vi "氨氮通讯.vi"() -> ()   [LabVIEW 2016, in "斯坦道氨氮.lvlib"]
uses:
  <vilib>/Plasmionique/MB Master/MB_Master_TCP/MB_Master_TCP.lvclass
  C:/Program Files (x86)/National Instruments/LabVIEW 2016/vi.lib/Plasmionique/MB Master/MB_Master/MB_Master.lvclass
  <vilib>/NI/Modbus Library/API/Wrapper/Create TCP Slave.vi
  <vilib>/Utility/config.llb/Write Key (String).vi
  <vilib>/Plasmionique/MB Master/MB_Master/MB_Master.lvclass
  <vilib>/NI/Modbus Library/API/slave/Modbus Slave.lvclass
  <vilib>/Utility/config.llb/NI_LVConfig.lvlib
  <vilib>/Plasmionique/MB Master/MB Master.lvlib
  <vilib>/NI/Modbus Library/API/Wrapper/API Main.lvlib
panel:
  out "测量数据区":T1 {"单位" items=["ug/L", "mg/L", "ppm", "mg/m3", "cm", "ppb", "ug/m3", "%", "nmol/mol", "umol/mol", "MPN/L", "MPN/100ml", "ng/m3", "NTU", "无量纲", "ms/cm", "us/cm", "℃", "mV", "万个/L"]}
  out "状态告警区":u16[](array[numeric])
  out "测量数据区":u16[](array[numeric])
  out "序列号":string
  out "状态告警区":T2
  out "status":bool
  out "关键参数区":T3
  in  "读关键参数区":bool
  in  "读状态告警区":bool
  in  "读测量数据区":bool
  in  "站号":u16(ring) items=["总磷"=1, "氨氮"=3]
  in  "停止":bool
  in  "启动":bool
  in  "控制命令":u16(ring) items=["启动测量"=1, "标样核查"=2, "零点核查"=3, "跨度核查"=4, "空白测试"=5, "平行样测试"=6, "加标回收"=7, "空白校准"=8, "标样校准"=9, "初始化（清洗）"=10, "停止测试"=11, "仪器重启"=12, "校时"=13, "模式设置"=14, "测量间隔设置"=15]
  in  "控制命令参数":u16[](array[numeric]) format="%04xH"
  in  "VISA Resource":refnum<visa-resource-name>
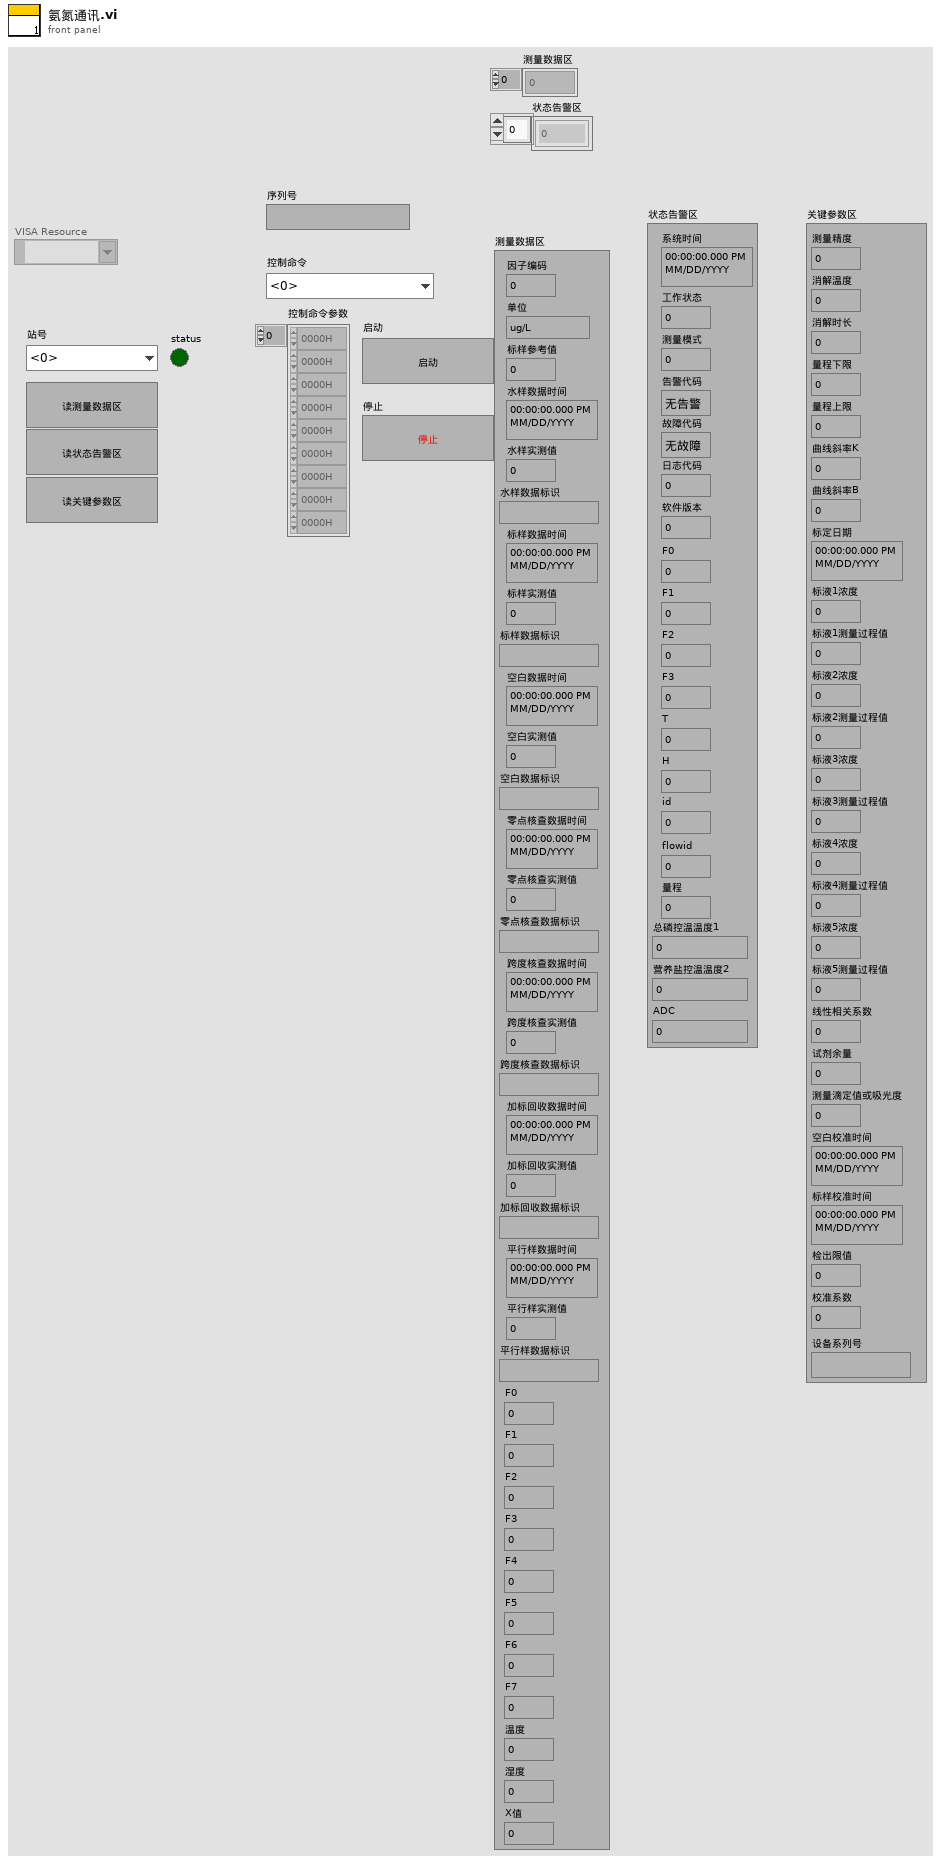
[diagram p1: front panel]
types:
  T1 = cluster{"因子编码":u32, "单位":u16, "标样参考值":sgl, "水样数据时间":timestamp, "水样实测值":sgl, "水样数据标识":string, "标样数据时间":timestamp, "标样实测值":sgl, "标样数据标识":string, "空白数据时间":timestamp, "空白实测值":sgl, "空白数据标识":string, "零点核查数据时间":timestamp, "零点核查实测值":sgl, "零点核查数据标识":string, "跨度核查数据时间":timestamp, "跨度核查实测值":sgl, "跨度核查数据标识":string, "加标回收数据时间":timestamp, "加标回收实测值":sgl, "加标回收数据标识":string, "平行样数据时间":timestamp, "平行样实测值":sgl, "平行样数据标识":string, "F0":sgl, "F1":sgl, "F2":sgl, "F3":sgl, "F4":sgl, "F5":sgl, "F6":sgl, "F7":sgl, "温度":sgl, "湿度":sgl, "X值":sgl}
  T2 = cluster{"系统时间":timestamp, "工作状态":u16, "测量模式":u16, "告警代码":enum16{"无告警", "缺试剂告警", "缺水样告警", "缺蒸馏水告警", "缺标液告警", "仪表漏液告警", "标定异常告警", "超量程告警", "加热异常", "低试剂预警", "超上限告警", "超下限告警", "仪表内部其他异常", "滴定异常告警", "电极异常告警", "量程切换告警", "参数设置告警", "PH电极电位异常", "电导率电极异常", "浊度光度异常", "溶解氧电极异常", "溶解氧光强异常", "温度异常告警", "PH异常告警", "溶解氧异常告警", "电导率异常告警", "浊度异常告警", "叶绿素异常告警", "藻密度异常告警", "蓝绿藻异常告警", "ORP异常告警", "氨氮异常告警", "清洁刷异常告警", "SD卡异常告警", "蓝牙异常告警", "Wifi异常告警", "流程异常告警"}, "故障代码":enum16{"无故障", "电机故障", "温度故障", "通讯故障", "滴定故障"}, "日志代码":u16, "软件版本":u16, "F0":sgl, "F1":sgl, "F2":sgl, "F3":sgl, "T":sgl, "H":sgl, "id":u16, "flowid":u16, "量程":u16, "ADC":sgl, "营养盐控温温度2":sgl, "总磷控温温度1":sgl}
  T3 = cluster{"测量精度":u16, "消解温度":u16, "消解时长":u16, "量程下限":sgl, "量程上限":sgl, "曲线斜率K":sgl, "曲线斜率B":sgl, "标定日期":timestamp, "标液1浓度":sgl, "标液1测量过程值":sgl, "标液2浓度":sgl, "标液2测量过程值":sgl, "标液3浓度":sgl, "标液3测量过程值":sgl, "标液4浓度":sgl, "标液4测量过程值":sgl, "标液5浓度":sgl, "标液5测量过程值":sgl, "线性相关系数":sgl, "试剂余量":u32, "测量滴定值或吸光度":sgl, "空白校准时间":timestamp, "标样校准时间":timestamp, "检出限值":sgl, "校准系数":sgl, "设备系列号":string}
  T4 = typedef "NI_LVConfig.lvlib/Config Data RefNum.ctl" = refnum<k1>
  T5 = enum8{"Enabled", "Disabled", "Disabled and Grayed Out"}
  T6 = cluster{"系统时间":timestamp, "工作状态":enum16{"空闲", "水样测试", "标样核查", "零点核查", "跨度核查", "空白测试", "平行样测试", "加标回收", "空白校准", "标样校准", "初始化（清洗）"}, "测量模式":enum16{"待机", "连续模式", "周期模式", "定点模式", "受控模式", "手动模式"}, "告警代码":enum16{"无告警", "缺试剂告警", "缺水样告警", "缺蒸馏水告警", "缺标液告警", "仪表漏液告警", "标定异常告警", "超量程告警", "加热异常", "低试剂预警", "超上限告警", "超下限告警", "仪表内部其他异常", "滴定异常告警", "电极异常告警", "量程切换告警", "参数设置告警", "PH电极电位异常", "电导率电极异常", "浊度光度异常", "溶解氧电极异常", "溶解氧光强异常", "温度异常告警", "PH异常告警", "溶解氧异常告警", "电导率异常告警", "浊度异常告警", "叶绿素异常告警", "藻密度异常告警", "蓝绿藻异常告警", "ORP异常告警", "氨氮异常告警", "清洁刷异常告警", "SD卡异常告警", "蓝牙异常告警", "Wifi异常告警", "流程异常告警"}, "故障代码":enum16{"无故障", "电机故障", "温度故障", "通讯故障", "滴定故障"}, "日志代码":u16, "软件版本":u16, "F0":sgl, "F1":sgl, "F2":sgl, "F3":sgl, "T":sgl, "H":sgl, "id":u16, "flowid":u16, "量程":u16, "总磷控温温度1":sgl, "营养盐控温温度2":sgl, "ADC":sgl}
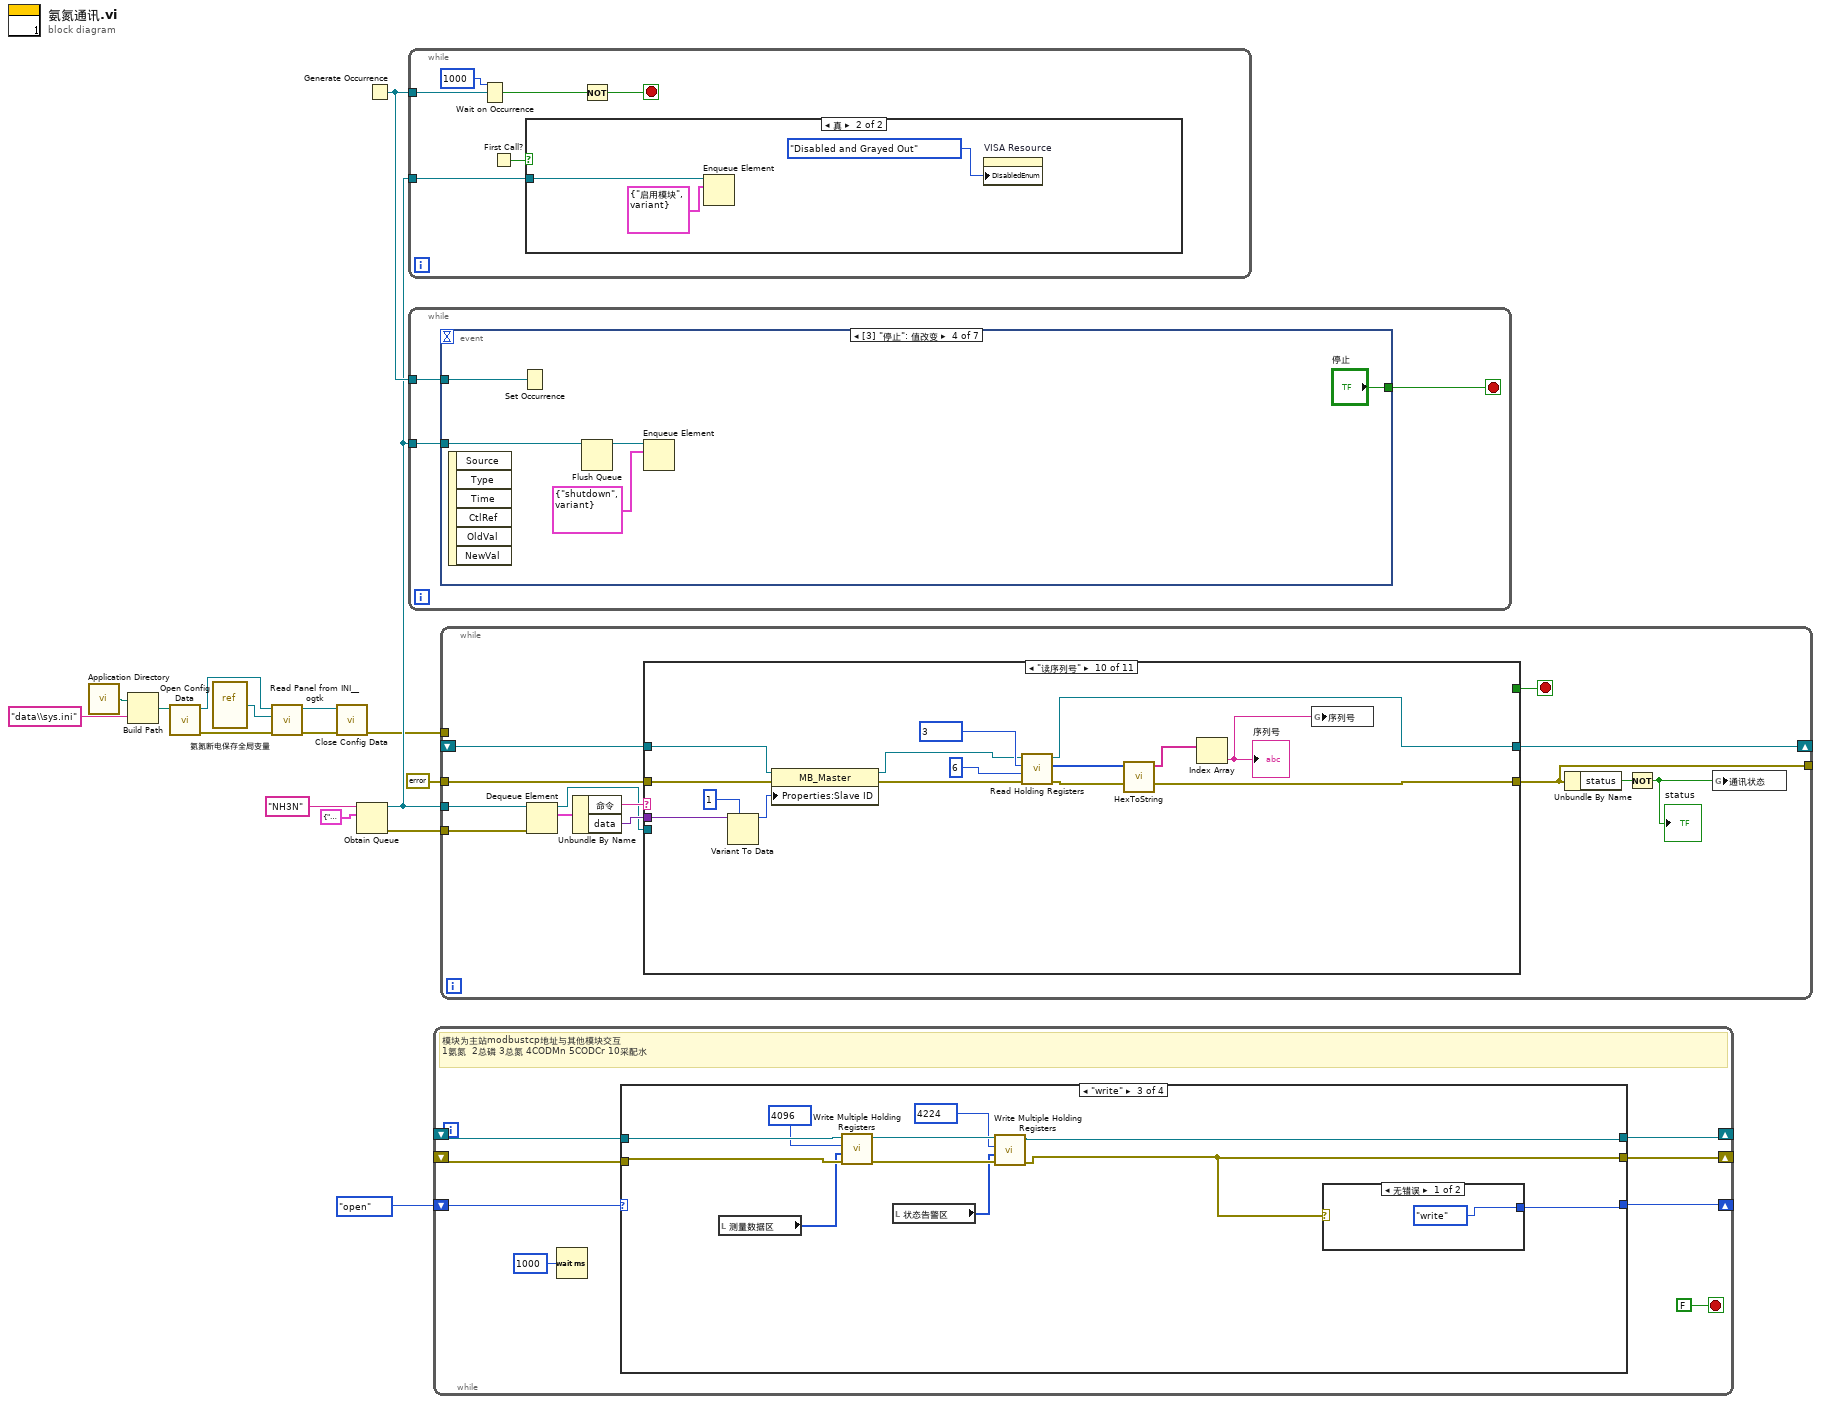
[diagram p0: block diagram]
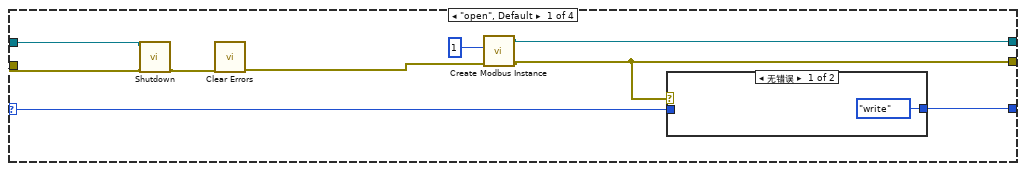
[diagram p2: hidden frame]
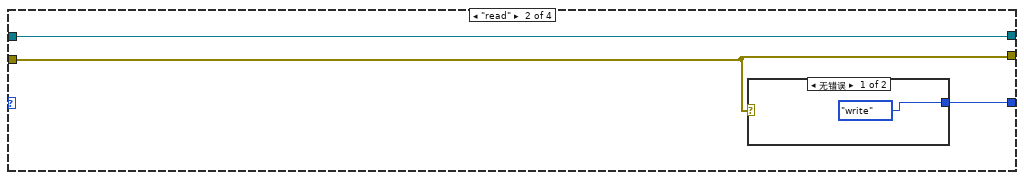
[diagram p4: hidden frame]
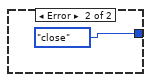
[diagram p5: hidden frame]
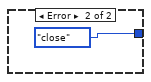
[diagram p6: hidden frame]
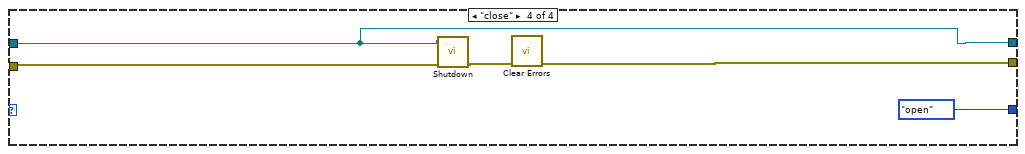
[diagram p7: hidden frame]
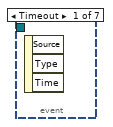
[diagram p9: hidden frame]
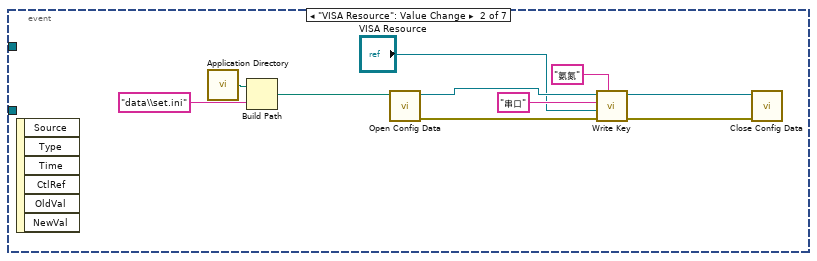
[diagram p10: hidden frame]
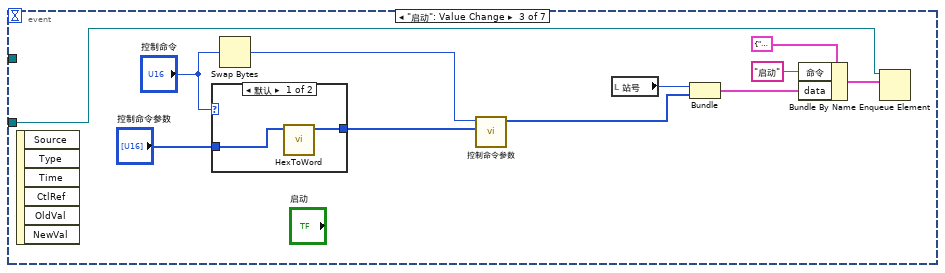
[diagram p11: hidden frame]
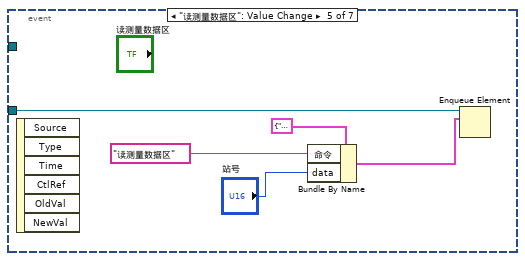
[diagram p13: hidden frame]
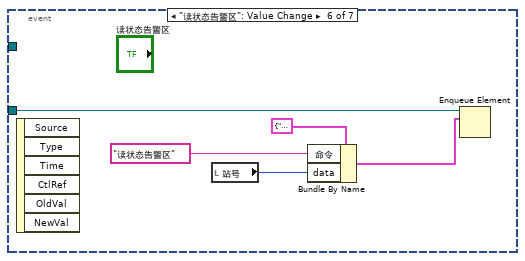
[diagram p14: hidden frame]
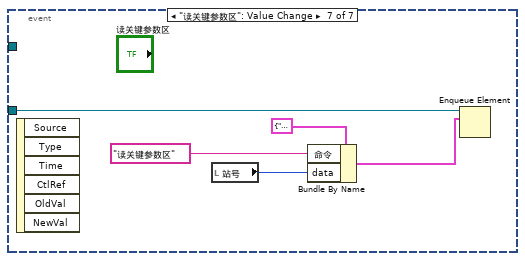
[diagram p15: hidden frame]
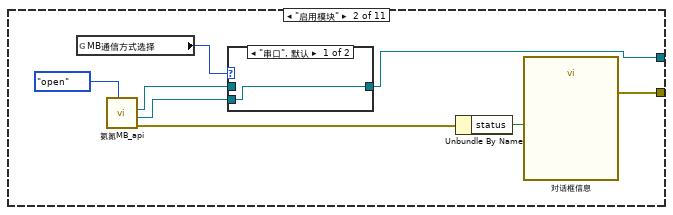
[diagram p17: hidden frame]
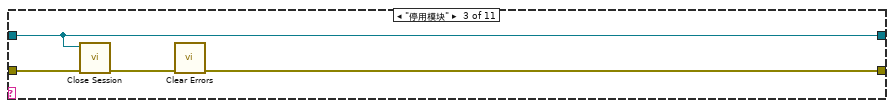
[diagram p19: hidden frame]
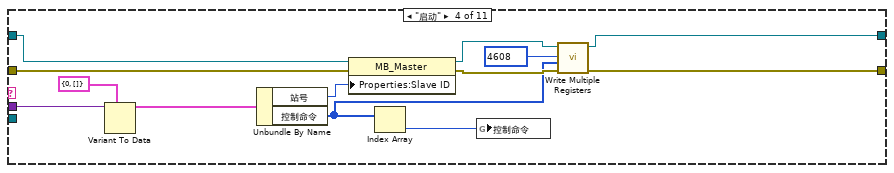
[diagram p20: hidden frame]
diagram:
  n1 = call <vilib>:"Application Directory.vi"() -> ("Application Directory"=w3:path)
  n2 = Build Path(base path=w3, name or relative path="data\\sys.ini" ("名称或相对路径")) -> (appended path=w5:path)
  n3 = call <vilib>:"Open Config Data.vi"("configuration file path"=w5) -> ("error out"=w9:errorcluster, "refnum"=w6:T4)  [unwired: 8 in, 1 out]
  n4 = vi-ref "氨氮断电保存全局变量.vi"() -> (w7:refnum<vi>)
  n5 = call <userlib>:"Read Panel from INI__ogtk.vi"("error in (no error)"=w9, "VI ref"=w7, "refnum"=w6) -> ("error out"=w10:errorcluster, "refnum out"=w8:T4)  [unwired: 7 in]
  n6 = call <vilib>:"Close Config Data.vi"("error in (no error)"=w10, "refnum"=w8) -> ("error out"=w2:errorcluster)  [unwired: 8 in, 1 out]
  n7 = Obtain Queue(name (unnamed)="NH3N" ("名称（未命名）"), element data type=cluster{"命令":string, "data":variant} {"命令"="", "data"=variant}) -> (queue out=w11:refnum<queue>, error out=w14:errorcluster)  [unwired: 3 in, 1 out]
  n8 = Generate Occurrence() -> (w12:refnum<k4>)
  n9 = while {
    tunnel: w12 -> [w22]
    tunnel: w11 -> [w18]
    stop <- w19 stop-if-true
    n10 = Wait on Occurrence(2:w22, 3:1000 ("毫秒超时(-1)")) -> (0:w20:bool)  [unwired: 1 in]
    n11 = First Call?() -> (First Call?: T/F=w17:bool)
    n12 = case shown="真" w17 {
      tunnel: w18 -> [_ w24]
      frame False {
      }
      frame True {
        n13 = Enqueue Element(queue=w24, element=cluster{"命令":string, "data":variant} {"命令"="启用模块", "data"=variant} ("元素")) -> ()  [unwired: 2 in, 3 out]
        n14 = property on="VISA Resource" class="VISAName"("DisabledEnum"=T5."Disabled and Grayed Out" ("禁用")) -> ()  [unwired: 2 in, 2 out]
      }
    }
    n15 = Not(x=w20) -> (.not. x?=w19:bool)
  }
  n16 = while {
    tunnel: w11 -> [w28]
    tunnel: w12 -> [w26]
    stop <- w27 stop-if-true
    n17 = event shown="[3] \"停止\": 值改变" {
      selector: _ -> [_ _ _ _ _ _ _]
      dyn-events: _ -> [_ _ _ _ _ _ _]
      timeout: _ -> [_ _ _ _ _ _ _]
      tunnel: w28 -> [_ _ w49 w56 w62 w67 w72]
      tunnel: [_ _ _ "停止" _ _ _] -> w27
      tunnel: w26 -> [_ _ _ w53 _ _ _]
      event Timeout {
        n18 = event-data() -> ()  [unwired: 1 in, 3 out]
      }
      event "VISA Resource": Value Change {
        n19 = event-data() -> ()  [unwired: 1 in, 6 out]
        n20 = call <vilib>:"Application Directory.vi"() -> ("Application Directory"=w31:path)
        n21 = Build Path(base path=w31, name or relative path="data\\set.ini" ("名称或相对路径")) -> (appended path=w32:path)
        n22 = call <vilib>:"Open Config Data.vi"("configuration file path"=w32) -> ("error out"=w38:errorcluster, "refnum"=w37:T4)  [unwired: 8 in, 1 out]
        n23 = call-poly <vilib>:"Write Key.vi"("section"="氨氮", "error in (no error)"=w38, "value"="VISA Resource", "key"="串口", "refnum"=w37) -> ("error out"=w34:errorcluster, "refnum out"=w30:T4)  [unwired: 4 in, 1 out]
        n24 = call <vilib>:"Close Config Data.vi"("error in (no error)"=w34, "refnum"=w30) -> ()  [unwired: 8 in, 2 out]
      }
      event "启动": Value Change {
        n25 = event-data() -> ()  [unwired: 1 in, 6 out]
        n26 = case shown="默认" "控制命令" {
          tunnel: "控制命令参数" -> [w51 w52]
          tunnel: [w50 w52] -> w39
          frame Default {
            n27 = call "HexToWord.vi"("数组"=w51) -> ("WORD"=w50:u16[])  [unwired: 10 in]
          }
          frame 13 {
          }
        }
        n28 = Swap Bytes(anything="控制命令") -> (byte swapped=w42:u16)
        n29 = call "控制命令参数.vi"("控制命令参数"=w39, "控制命令"=w42) -> ("控制命令输出"=w45:u16[])  [unwired: 9 in]
        n30 = local read "站号"() -> (w44:u16)
        n31 = Bundle("站号"=w44, "控制命令输出"=w45) -> (w43:cluster{"站号":u16, "控制命令输出":u16[]})  [unwired: 1 in]
        n32 = Bundle By Name(cluster=cluster{"命令":string, "data":variant} {"命令"="", "data"=variant} ("元素"), "命令"="启动", "data"=w43) -> (w47:cluster{"命令":string, "data":variant})
        n33 = Enqueue Element(queue=w49, element=w47) -> ()  [unwired: 2 in, 3 out]
      }
      event "停止": Value Change {
        n34 = event-data() -> ()  [unwired: 1 in, 6 out]
        n35 = Set Occurrence(w53) -> ()
        n36 = Flush Queue(queue=w56) -> (queue out=w55:refnum<queue>)  [unwired: 1 in, 2 out]
        n37 = Enqueue Element(queue=w55, element=cluster{"命令":string, "data":variant} {"命令"="shutdown", "data"=variant} ("元素")) -> ()  [unwired: 2 in, 3 out]
      }
      event "读测量数据区": Value Change {
        n38 = event-data() -> ()  [unwired: 1 in, 6 out]
        n39 = Bundle By Name(cluster=cluster{"命令":string, "data":variant} {"命令"="", "data"=variant} ("元素"), "命令"="读测量数据区", "data"="站号") -> (w60:cluster{"命令":string, "data":variant})
        n40 = Enqueue Element(queue=w62, element=w60) -> ()  [unwired: 2 in, 3 out]
      }
      event "读状态告警区": Value Change {
        n41 = event-data() -> ()  [unwired: 1 in, 6 out]
        n42 = local read "站号"() -> (w63:u16)
        n43 = Bundle By Name(cluster=cluster{"命令":string, "data":variant} {"命令"="", "data"=variant} ("元素"), "命令"="读状态告警区", "data"=w63) -> (w65:cluster{"命令":string, "data":variant})
        n44 = Enqueue Element(queue=w67, element=w65) -> ()  [unwired: 2 in, 3 out]
      }
      event "读关键参数区": Value Change {
        n45 = event-data() -> ()  [unwired: 1 in, 6 out]
        n46 = local read "站号"() -> (w68:u16)
        n47 = Bundle By Name(cluster=cluster{"命令":string, "data":variant} {"命令"="", "data"=variant} ("元素"), "命令"="读关键参数区", "data"=w68) -> (w70:cluster{"命令":string, "data":variant})
        n48 = Enqueue Element(queue=w72, element=w70) -> ()  [unwired: 2 in, 3 out]
      }
    }
  }
  n49 = while {
    shift-right: [w78] -> _
    shift-left: _ -> [w80]
    shift-right: [w77] -> _
    shift-left: _ -> [w79]
    shift-right: [w74] -> _
    shift-left: enum16{"open", "read", "write", "close"}."open" -> [w75]
    stop <- FALSE stop-if-true
    # "模块为主站modbustcp地址与其他模块交互\n1氨氮  2总磷 3总氮 4CODMn 5CODCr 10采配水"
    n50 = Wait (ms)(milliseconds to wait=u32 1000 ("等待时间（毫秒）")) -> ()  [unwired: 1 out]
    n51 = case shown="\"write\"" w75 {
      selector: w75 -> [w89 _ _ _]
      tunnel: w80 -> [w83 w92 w106 w112]
      tunnel: w79 -> [w82 w93 w105 w111]
      tunnel: [w86 w92 w101 w112] -> w78
      tunnel: [w85 w93 w100 w114] -> w77
      tunnel: [w88 w94 w107 enum16{"open", "read", "write", "close"}."open"] -> w74
      frame "open", Default {
        n52 = call-dynamic "Shutdown.vi"("error in"=w82, "Modbus slave in"=w83) -> ("error out"=w81:errorcluster)  [unwired: 9 in]
        n53 = call <vilib>:"Clear Errors.vi"("error in (no error)"=w81) -> ("error out"=w84:errorcluster)  [unwired: 5 in, 1 out]
        n54 = call-poly <vilib>:"Create Modbus Instance.vi"("error in"=w84, "port (502)"=u16 1) -> ("error out"=w85:errorcluster, "TCP slave instance"=w86:refnum<class "Modbus Slave.lvclass">)  [unwired: 8 in]
        n55 = case shown="无错误" w85 {
          tunnel: w89 -> [_ w91]
          tunnel: [enum16{"open", "read", "write", "close"}."write" w91] -> w88
          frame No Error {
          }
          frame Error {
          }
        }
      }
      frame "read" {
        n56 = case shown="无错误" w93 {
          tunnel: [enum16{"open", "read", "write", "close"}."write" enum16{"open", "read", "write", "close"}."close"] -> w94
          frame No Error {
          }
          frame Error {
          }
        }
      }
      frame "write" {
        n57 = local read "测量数据区"() -> (w99:u16[])
        n58 = call-dynamic "Write Multiple Holding Registers.vi"("error in"=w105, "registers to write"=w99, "starting address"=u16 4096, "Modbus slave in"=w106) -> ("error out"=w102:errorcluster, "Modbus slave out"=w103:refnum<class "Modbus Slave.lvclass">)  [unwired: 6 in]
        n59 = local read "状态告警区"() -> (w97:u16[])
        n60 = call-dynamic "Write Multiple Holding Registers.vi"("error in"=w102, "registers to write"=w97, "starting address"=u16 4224, "Modbus slave in"=w103) -> ("error out"=w100:errorcluster, "Modbus slave out"=w101:refnum<class "Modbus Slave.lvclass">)  [unwired: 6 in]
        n61 = case shown="无错误" w100 {
          tunnel: [enum16{"open", "read", "write", "close"}."write" enum16{"open", "read", "write", "close"}."close"] -> w107
          frame No Error {
          }
          frame Error {
          }
        }
      }
      frame "close" {
        n62 = call-dynamic "Shutdown.vi"("error in"=w111, "Modbus slave in"=w112) -> ("error out"=w110:errorcluster)  [unwired: 9 in]
        n63 = call <vilib>:"Clear Errors.vi"("error in (no error)"=w110) -> ("error out"=w114:errorcluster)  [unwired: 5 in, 1 out]
      }
    }
  }
  n64 = while {
    tunnel: w11 -> [w127]
    tunnel: w14 -> [w126]
    shift-right: [w124] -> _
    shift-left: _ -> [w123]
    tunnel: errorcluster {"status"=FALSE, "code"=0, "source"=""} ("error out") -> [w122]
    tunnel: [w117] -> _
    tunnel: w2 -> [_]
    stop <- w125 stop-if-true
    n65 = Dequeue Element(queue=w127, error in (no error)=w126) -> (queue out=w118:refnum<queue>, element=w120:cluster{"命令":string, "data":variant})  [unwired: 1 in, 2 out]
    n66 = Unbundle By Name(w120) -> ("命令"=w121:string, "data"=w119:variant)
    n67 = case shown="\"读序列号\"" w121 {
      tunnel: w119 -> [_ _ _ w153 w164 w181 w190 w200 w215 w229 _]
      tunnel: w118 -> [_ _ _ _ _ _ _ _ _ _ w242]
      tunnel: [_ _ _ _ _ _ _ _ _ _ TRUE] -> w125
      tunnel: [w128 w130 w140 w156 w167 w183 w195 w209 w222 w236 w238] -> w124
      tunnel: [w129 w136 w141 w155 w166 w182 w184 w210 w223 w237 w239] -> w117
      tunnel: w123 -> [w128 _ w140 w152 w163 w180 w189 w203 w218 w232 w238]
      tunnel: w122 -> [w129 _ w143 w149 w160 w177 w187 w204 w219 w233 w240]
      frame Default {
      }
      frame "启用模块" {
        n68 = global read "氨氮断电保存全局变量.vi" "MB通信方式选择"() -> (w133:enum16{"串口", "TCP"})
        n69 = call "氨氮MB_api.vi"("STEP"=enum16{"open", "read", "write", "close"}."open") -> ("error out"=w134:errorcluster, "MB session out"=w131:refnum<class "MB_Master.lvclass">, "MB_TCP session"=w132:refnum<class "MB_Master_TCP.lvclass">)  [unwired: 7 in, 1 out]
        n70 = case shown="\"串口\", 默认" w133 {
          tunnel: w132 -> [_ w139]
          tunnel: w131 -> [w138 _]
          tunnel: [w138 w139] -> w130
          frame "串口", Default {
          }
          frame "TCP" {
          }
        }
        n71 = Unbundle By Name(w134) -> ("status"=w137:bool)
        n72 = call "对话框信息"("Enable"=w137) -> ("error out"=w136:errorcluster)  [unwired: 9 in, 1 out]
      }
      frame "停用模块" {
        n73 = call-dynamic "Close Session.vi"("error in (no error)"=w143, "MB session in"=w140) -> ("error out"=w142:errorcluster)  [unwired: 9 in]
        n74 = call <vilib>:"Clear Errors.vi"("error in (no error)"=w142) -> ("error out"=w141:errorcluster)  [unwired: 5 in, 1 out]
      }
      frame "启动" {
        n75 = Variant To Data(type=cluster{"站号":u16, "控制命令":u16[]} {"站号"=0, "控制命令"=[]} ("输出簇"), Variant=w153) -> (data=w147:cluster{"站号":u16, "控制命令":u16[]})  [unwired: 1 in, 1 out]
        n76 = Unbundle By Name(w147) -> ("站号"=w146:u16, "控制命令"=w144:u16[])
        n77 = property class="MB_Master"(reference=w152, error in=w149, "Properties:Slave ID"=w146) -> (reference out=w151:refnum<class "MB_Master.lvclass">, error out=w150:errorcluster)
        n78 = Index Array(array=w144) -> (element=w145:u16)  [unwired: 1 in]
        n79 = global write "VAR氨氮全局变量.vi" "控制命令"(w145) -> ()
        n80 = call <vilib>:"Write Multiple Registers.vi"("error in (no error)"=w150, "values"=w144, "starting address"=u16 4608, "MB session in"=w151) -> ("error out"=w155:errorcluster, "MB session out"=w156:refnum<class "MB_Master.lvclass">)  [unwired: 6 in]
      }
      frame "盲样测试" {
        n81 = Variant To Data(type=0, Variant=w164) -> (data=w157:i32)  [unwired: 1 in, 1 out]
        n82 = property class="MB_Master"(reference=w163, error in=w160, "Properties:Slave ID"=w157) -> (reference out=w162:refnum<class "MB_Master.lvclass">, error out=w161:errorcluster)
        n83 = case shown="默认" w157 {
          tunnel: [u16[] [] ("values") u16[] [33539, 0] ("values") u16[] [23555, 0] ("values")] -> w159
          frame Default {
          }
          frame 1 {
            # "总磷盲样测试命令"
          }
          frame 3 {
            # "氨氮盲样测试"
          }
        }
        n84 = call <vilib>:"Write Multiple Registers.vi"("error in (no error)"=w161, "values"=w159, "starting address"=u16 24592, "MB session in"=w162) -> ("error out"=w166:errorcluster, "MB session out"=w167:refnum<class "MB_Master.lvclass">)  [unwired: 6 in]
      }
      frame "debug" {
        n85 = Variant To Data(type=cluster{"站号":u16, "控制命令":u16[]} {"站号"=0, "控制命令"=[]} ("输出簇"), Variant=w181) -> (data=w175:cluster{"站号":u16, "控制命令":u16[]})  [unwired: 1 in, 1 out]
        n86 = Unbundle By Name(w175) -> ("站号"=w174:u16, "控制命令"=w172:u16[])
        n87 = property class="MB_Master"(reference=w180, error in=w177, "Properties:Slave ID"=w174) -> (reference out=w179:refnum<class "MB_Master.lvclass">, error out=w178:errorcluster)
        n88 = Index Array(array=w172) -> (element=w173:u16)  [unwired: 1 in]
        n89 = global write "VAR氨氮全局变量.vi" "控制命令"(w173) -> ()
        n90 = call <vilib>:"Write Multiple Registers.vi"("error in (no error)"=w178, "values"=w172, "starting address"=u16 24594, "MB session in"=w179) -> ("error out"=w182:errorcluster, "MB session out"=w183:refnum<class "MB_Master.lvclass">)  [unwired: 6 in]
      }
      frame "读测量数据区" {
        n91 = Variant To Data(type=u8 1 ("Slave ID"), Variant=w190) -> (data=w191:u8)  [unwired: 1 in, 1 out]
        n92 = property class="MB_Master"(reference=w189, error in=w187, "Properties:Slave ID"=w191) -> (reference out=w188:refnum<class "MB_Master.lvclass">, error out=w186:errorcluster)
        n93 = call <vilib>:"Read Holding Registers.vi"("error in (no error)"=w186, "quantity"=u16 83, "starting address"=u16 4096, "MB session in"=w188) -> ("error out"=w184:errorcluster, "Registers"=w185:u16[], "MB session out"=w195:refnum<class "MB_Master.lvclass">)  [unwired: 5 in]
        n94 = case shown="无错误" w184 {
          tunnel: w185 -> [w197 _]
          frame No Error {
            n95 = call "测量数据区.vi"("数组"=w197) -> ("测量数据区"=w196:T1)  [unwired: 10 in]
            "测量数据区" <- w196
            n96 = global write "VAR氨氮全局变量.vi" "测量数据区"(w196) -> ()
            "测量数据区" <- w197
          }
          frame Error {
          }
        }
      }
      frame "读状态告警区" {
        n97 = Variant To Data(type=u8 1 ("Slave ID"), Variant=w200) -> (data=w205:u8)  [unwired: 1 in, 1 out]
        n98 = property class="MB_Master"(reference=w203, error in=w204, "Properties:Slave ID"=w205) -> (reference out=w202:refnum<class "MB_Master.lvclass">, error out=w201:errorcluster)
        n99 = call <vilib>:"Read Holding Registers.vi"("error in (no error)"=w201, "quantity"=u16 24, "starting address"=u16 4224, "MB session in"=w202) -> ("error out"=w210:errorcluster, "Registers"=w199:u16[], "MB session out"=w209:refnum<class "MB_Master.lvclass">)  [unwired: 5 in]
        "状态告警区" <- w199
        n100 = call "状态告警区.vi"("数组"=w199) -> ("状态告警区"=w198:T6)  [unwired: 10 in]
        "状态告警区" <- w198
        n101 = global write "VAR氨氮全局变量.vi" "状态告警区"(w198) -> ()
      }
      frame "读关键参数区" {
        n102 = Variant To Data(type=u8 1 ("Slave ID"), Variant=w215) -> (data=w213:u8)  [unwired: 1 in, 1 out]
        n103 = property class="MB_Master"(reference=w218, error in=w219, "Properties:Slave ID"=w213) -> (reference out=w217:refnum<class "MB_Master.lvclass">, error out=w216:errorcluster)
        n104 = call <vilib>:"Read Holding Registers.vi"("error in (no error)"=w216, "quantity"=u16 19, "starting address"=u16 4256, "MB session in"=w217) -> ("error out"=w223:errorcluster, "Registers"=w212:u16[], "MB session out"=w222:refnum<class "MB_Master.lvclass">)  [unwired: 5 in]
        n105 = call "关键参数区.vi"("数组"=w212) -> ("关键参数区"=w211:T3)  [unwired: 10 in]
        "关键参数区" <- w211
        n106 = global write "VAR氨氮全局变量.vi" "关键参数区"(w211) -> ()
      }
      frame "读序列号" {
        n107 = Variant To Data(type=u8 1 ("Slave ID"), Variant=w229) -> (data=w227:u8)  [unwired: 1 in, 1 out]
        n108 = property class="MB_Master"(reference=w232, error in=w233, "Properties:Slave ID"=w227) -> (reference out=w231:refnum<class "MB_Master.lvclass">, error out=w230:errorcluster)
        n109 = call <vilib>:"Read Holding Registers.vi"("error in (no error)"=w230, "quantity"=u16 6, "starting address"=u16 3, "MB session in"=w231) -> ("error out"=w237:errorcluster, "Registers"=w226:u16[], "MB session out"=w236:refnum<class "MB_Master.lvclass">)  [unwired: 5 in]
        n110 = call "HexToString.vi"("数组"=w226) -> ("STRING"=w225:string[])  [unwired: 10 in]
        n111 = Index Array(array=w225) -> (element=w224:string)  [unwired: 1 in]
        "序列号" <- w224
        n112 = global write "VAR氨氮全局变量.vi" "序列号"(w224) -> ()
      }
      frame "shutdown" {
        n113 = call-dynamic "Close Session.vi"("error in (no error)"=w240, "MB session in"=w238) -> ("error out"=w239:errorcluster)  [unwired: 9 in]
        n114 = Flush Queue(queue=w242) -> (queue out=w241:refnum<queue>)  [unwired: 1 in, 2 out]
        n115 = Release Queue(queue=w241) -> ()  [unwired: 2 in, 3 out]
      }
    }
    n116 = Unbundle By Name(w117) -> ("status"=w116:bool)
    n117 = Not(x=w116) -> (.not. x?=w115:bool)
    "status" <- w115
    n118 = global write "VAR氨氮全局变量.vi" "通讯状态"(w115) -> ()
  }
